vi "MissionControl2017.vi"() -> ()   [LabVIEW 2015, in "MissionControl2017.lvlib"]
uses:
  MissionControl2017.lvlib
  PathfindingSettings.ctl
  MovementSettings.ctl
  PathCostWeights.ctl
  IntermediatePositionGrids.ctl
  <vilib>/Utility/miscctls.llb/LVPoint32TypeDef.ctl
  LocalizationStatus.ctl
  <vilib>/Utility/miscctls.llb/LVBoundsTypeDef.ctl
  Vector.ctl
  PathOfMoves.ctl
  Move.ctl
  Overlord2017.lvlib
  Navigation2017.lvlib
  Navigation2017-util.lvlib
panel:
  in  "reset timer":bool
  out "millisecond timer value":u32
  in  "Turning Width (used in movement control)":dbl(slide)=0.1318325449365179 scale=0.05..0.5
  out "Waveform Chart 2":dbl(graph)=0.5
  out "Waveform Chart":dbl(graph)=0.5
  out "Motor PWM XY Graph":cluster{"X":dbl, "Y":dbl}[](graph)
  out "Position at Start of Pathfinding Calculation":T1={"x"=2.4736536245406993, "y"=1.8255455643190823, "angle"=3.0398193796851833, "valid"=TRUE, "lastUpdatedTime"=1416276.0}
  out "Current Localization Status (As Drawn Above)":T1={"x"=2.723915333589265, "y"=2.6113036938119802, "angle"=2.982809442272849, "valid"=TRUE, "lastUpdatedTime"=538657016.0}
  in  "Debug Mining":bool=TRUE
  in  "Debug Wheel Motors":bool
  out "navDebugBotSpin":dbl=1.1780972450961724
  out "y (m)":dbl=0.0073828125
  out "x (m)":dbl=3.51288
  in  "Debug Localization - Mouse":bool
  out "Mouse Wheel Sum":dbl
  out "Mouse Wheel Delta":i32
  out "Mouse Down Button":u16=1
  out "Mouse Coords":T2={"Horizontal"=524, "Vertical"=1}
  out "Mouse Down Coords":T2={"Horizontal"=778, "Vertical"=441}
  out "CurrMiningRun":i16(slide)=2 scale=0.0..3.0
  out "CurrStage":string="Moving to Mining Area"
  out "UsedDesperation":bool
  out "SpecifyingEndAngle":bool
  out "NextPointIsDestination":bool
  out "CurrNavStage":string="Waiting for localization..."
  out "FPS Indicator":bool
  in  "Pathfinding Settings":T3={"Movement Settings"={"Arrival Tolerance (m)"=0.01, "Closeness Threshold (m)"=0.5, "Pit Obstacle Radius (m)"=0.5, "Pit Locations"=[]}, "Dead Zone"=0.75, "Max Moves"=2.0, "Move Segment Length (m)"=0.2, "Path Cost Weights"={"Length Weight"=1.0, "Angle Weight"=0.0, "Angle Error Weight"=1000.0, "Angle Error Threshold"=0.314, "Per Move Penalty"=0.05, "Closeness Weight"=100.0, "Too Short Penalty"=100.0, "Too Short Threshold"=1.5}, "Desperation - Reduction Per Attempt (Ratio)"=0.9, "Desperation - Max Attempts"=1, "Log All Move Points"=TRUE, "Intermediate Position Grids"=[{"x1"=0.0, "x2"=1.75, "resolution"=0.15}, {"x1"=1.75, "x2"=7.38, "resolution"=0.4}]}
  out "Arena Pixel Size":i16[](array[numeric])=[1000, 512]
  out "Arena Control":picture
  # "NOTE: Open and pin\n\nMineOrDumpBlocking.vi\nand\nSetWheelMotorPWM.vi\n\nalongside when debugging."
  # "(Spin robot with arrow keys)"
  # "To toggle localization debugging:\n- Flip this switch <---\n- Set the Project Property -> Conditional Compilation Property\n\"DISCONNECT_LOCALIZATION\" to True or False"
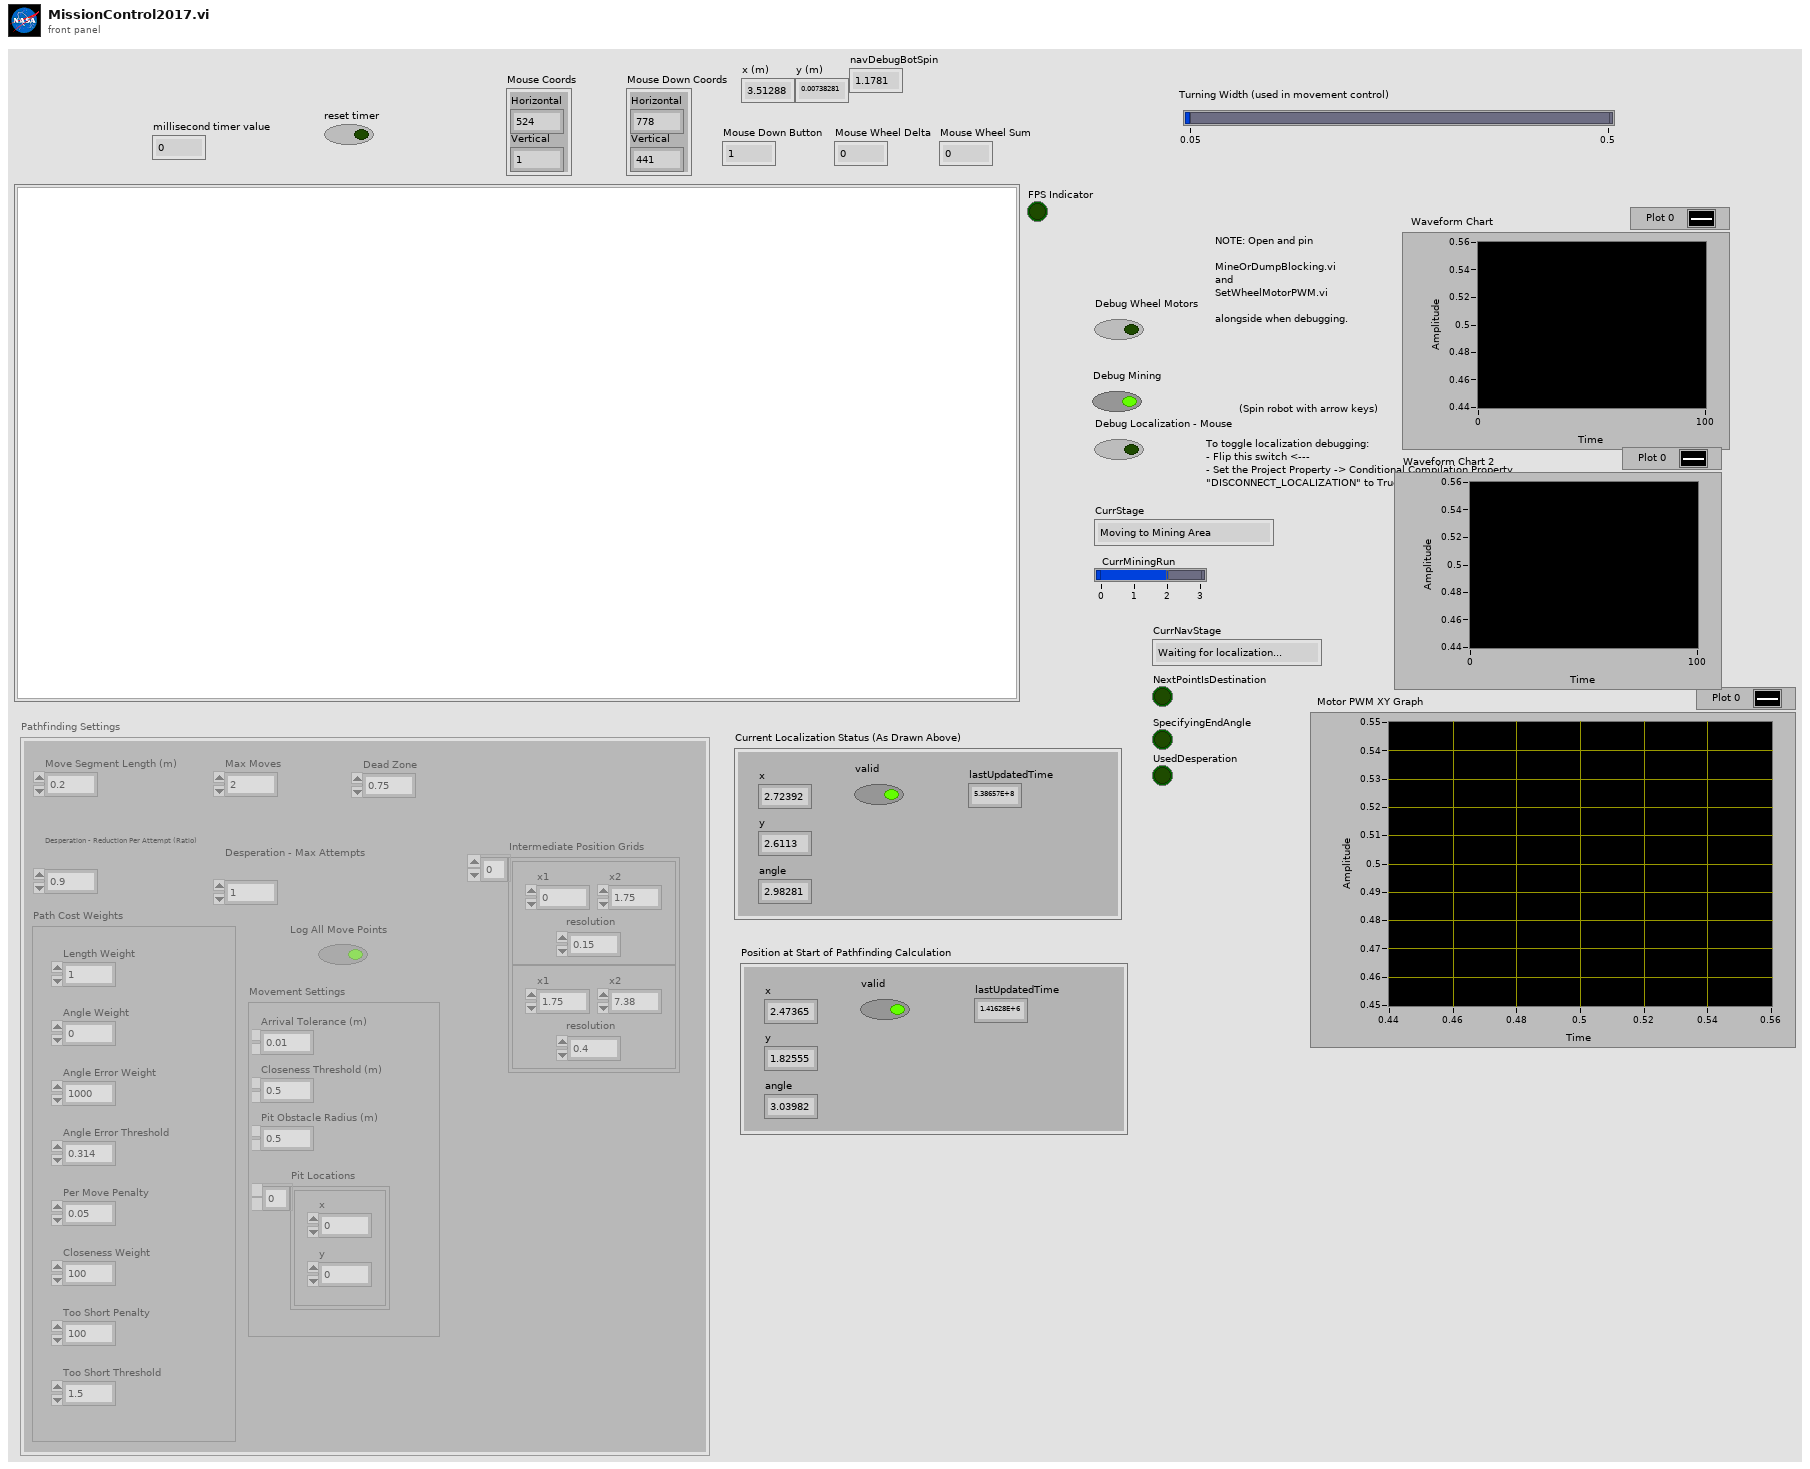
[diagram p1: front panel]
types:
  T1 = typedef "LocalizationStatus.ctl" = cluster{"x":dbl, "y":dbl, "angle":dbl, "valid":bool, "lastUpdatedTime":dbl}
  T2 = typedef "LVPoint32TypeDef.ctl" = cluster{"Horizontal":i32, "Vertical":i32}
  T3 = typedef "Navigation2017.lvlib/PathfindingSettings.ctl" = cluster{"Movement Settings":T4, "Dead Zone":dbl, "Max Moves":dbl, "Move Segment Length (m)":dbl, "Path Cost Weights":T5, "Desperation - Reduction Per Attempt (Ratio)":dbl, "Desperation - Max Attempts":i16, "Log All Move Points":bool, "Intermediate Position Grids":T6}
  T4 = typedef "Navigation2017.lvlib/MovementSettings.ctl" = cluster{"Arrival Tolerance (m)":dbl, "Closeness Threshold (m)":dbl, "Pit Obstacle Radius (m)":dbl, "Pit Locations":cluster{"x":dbl, "y":dbl}[]}
  T5 = typedef "Navigation2017.lvlib/PathCostWeights.ctl" = cluster{"Length Weight":dbl, "Angle Weight":dbl, "Angle Error Weight":dbl, "Angle Error Threshold":dbl, "Per Move Penalty":dbl, "Closeness Weight":dbl, "Too Short Penalty":dbl, "Too Short Threshold":dbl}
  T6 = typedef "Navigation2017.lvlib/IntermediatePositionGrids.ctl" = cluster{"x1":dbl, "x2":dbl, "resolution":dbl}[]
  T7 = typedef "LVBoundsTypeDef.ctl" = cluster{"Width":u32, "Height":u32}
  T8 = typedef "eventvkey.ctl" = enum16{"ASCII", "Enter", "Return", "Shift", "Ctrl", "Alt", "Cmd", "Opt", "Caps", "NumLock", "Clear", "Break", "Up", "Down", "Left", "Right", "Insert", "Delete", "Home", "End", "PageUp", "PageDown", "Escape", "Help", "Pause", "ScrollLock", "F1", "F2", "F3", "F4", "F5", "F6", "F7", "F8", "F9", "F10", "F11", "F12", "F13", "F14", "F15", "F16", "F17", "F18", "F19", "F20", "F21", "F22", "F23", "F24", "Play", "VolumeUp", "VolumeDown", "Mute", "Two Byte Char"}
  T9 = typedef "imagedata.ctl" = cluster{"image type":i32, "image depth":i32, "image":u8[], "mask":u8[], "colors":u32[], "Rectangle":cluster{"left":i16, "top":i16, "right":i16, "bottom":i16}}
  T10 = typedef "Navigation2017.lvlib/Vector.ctl" = cluster{"x":dbl, "y":dbl, "angle":dbl}
  T11 = cluster{"Width":u16, "Style":enum32{"Solid", "Dash", "Dot", "DashDot", "DashDotDot"}}
  T12 = typedef "Navigation2017.lvlib/PathOfMoves.ctl" = cluster{"Dest Angle Error":dbl, "Dest Angle Considered":bool, "Moves":T13[]}
  T13 = typedef "Navigation2017.lvlib/Move.ctl" = cluster{"Did Reach Dest":bool, "Did Collide":bool, "Sum of Angle Changes (rad)":dbl, "Move Length (m)":dbl, "Closeness Sum":dbl, "Positions Along Move":T10[], "Moved Fwd":bool}
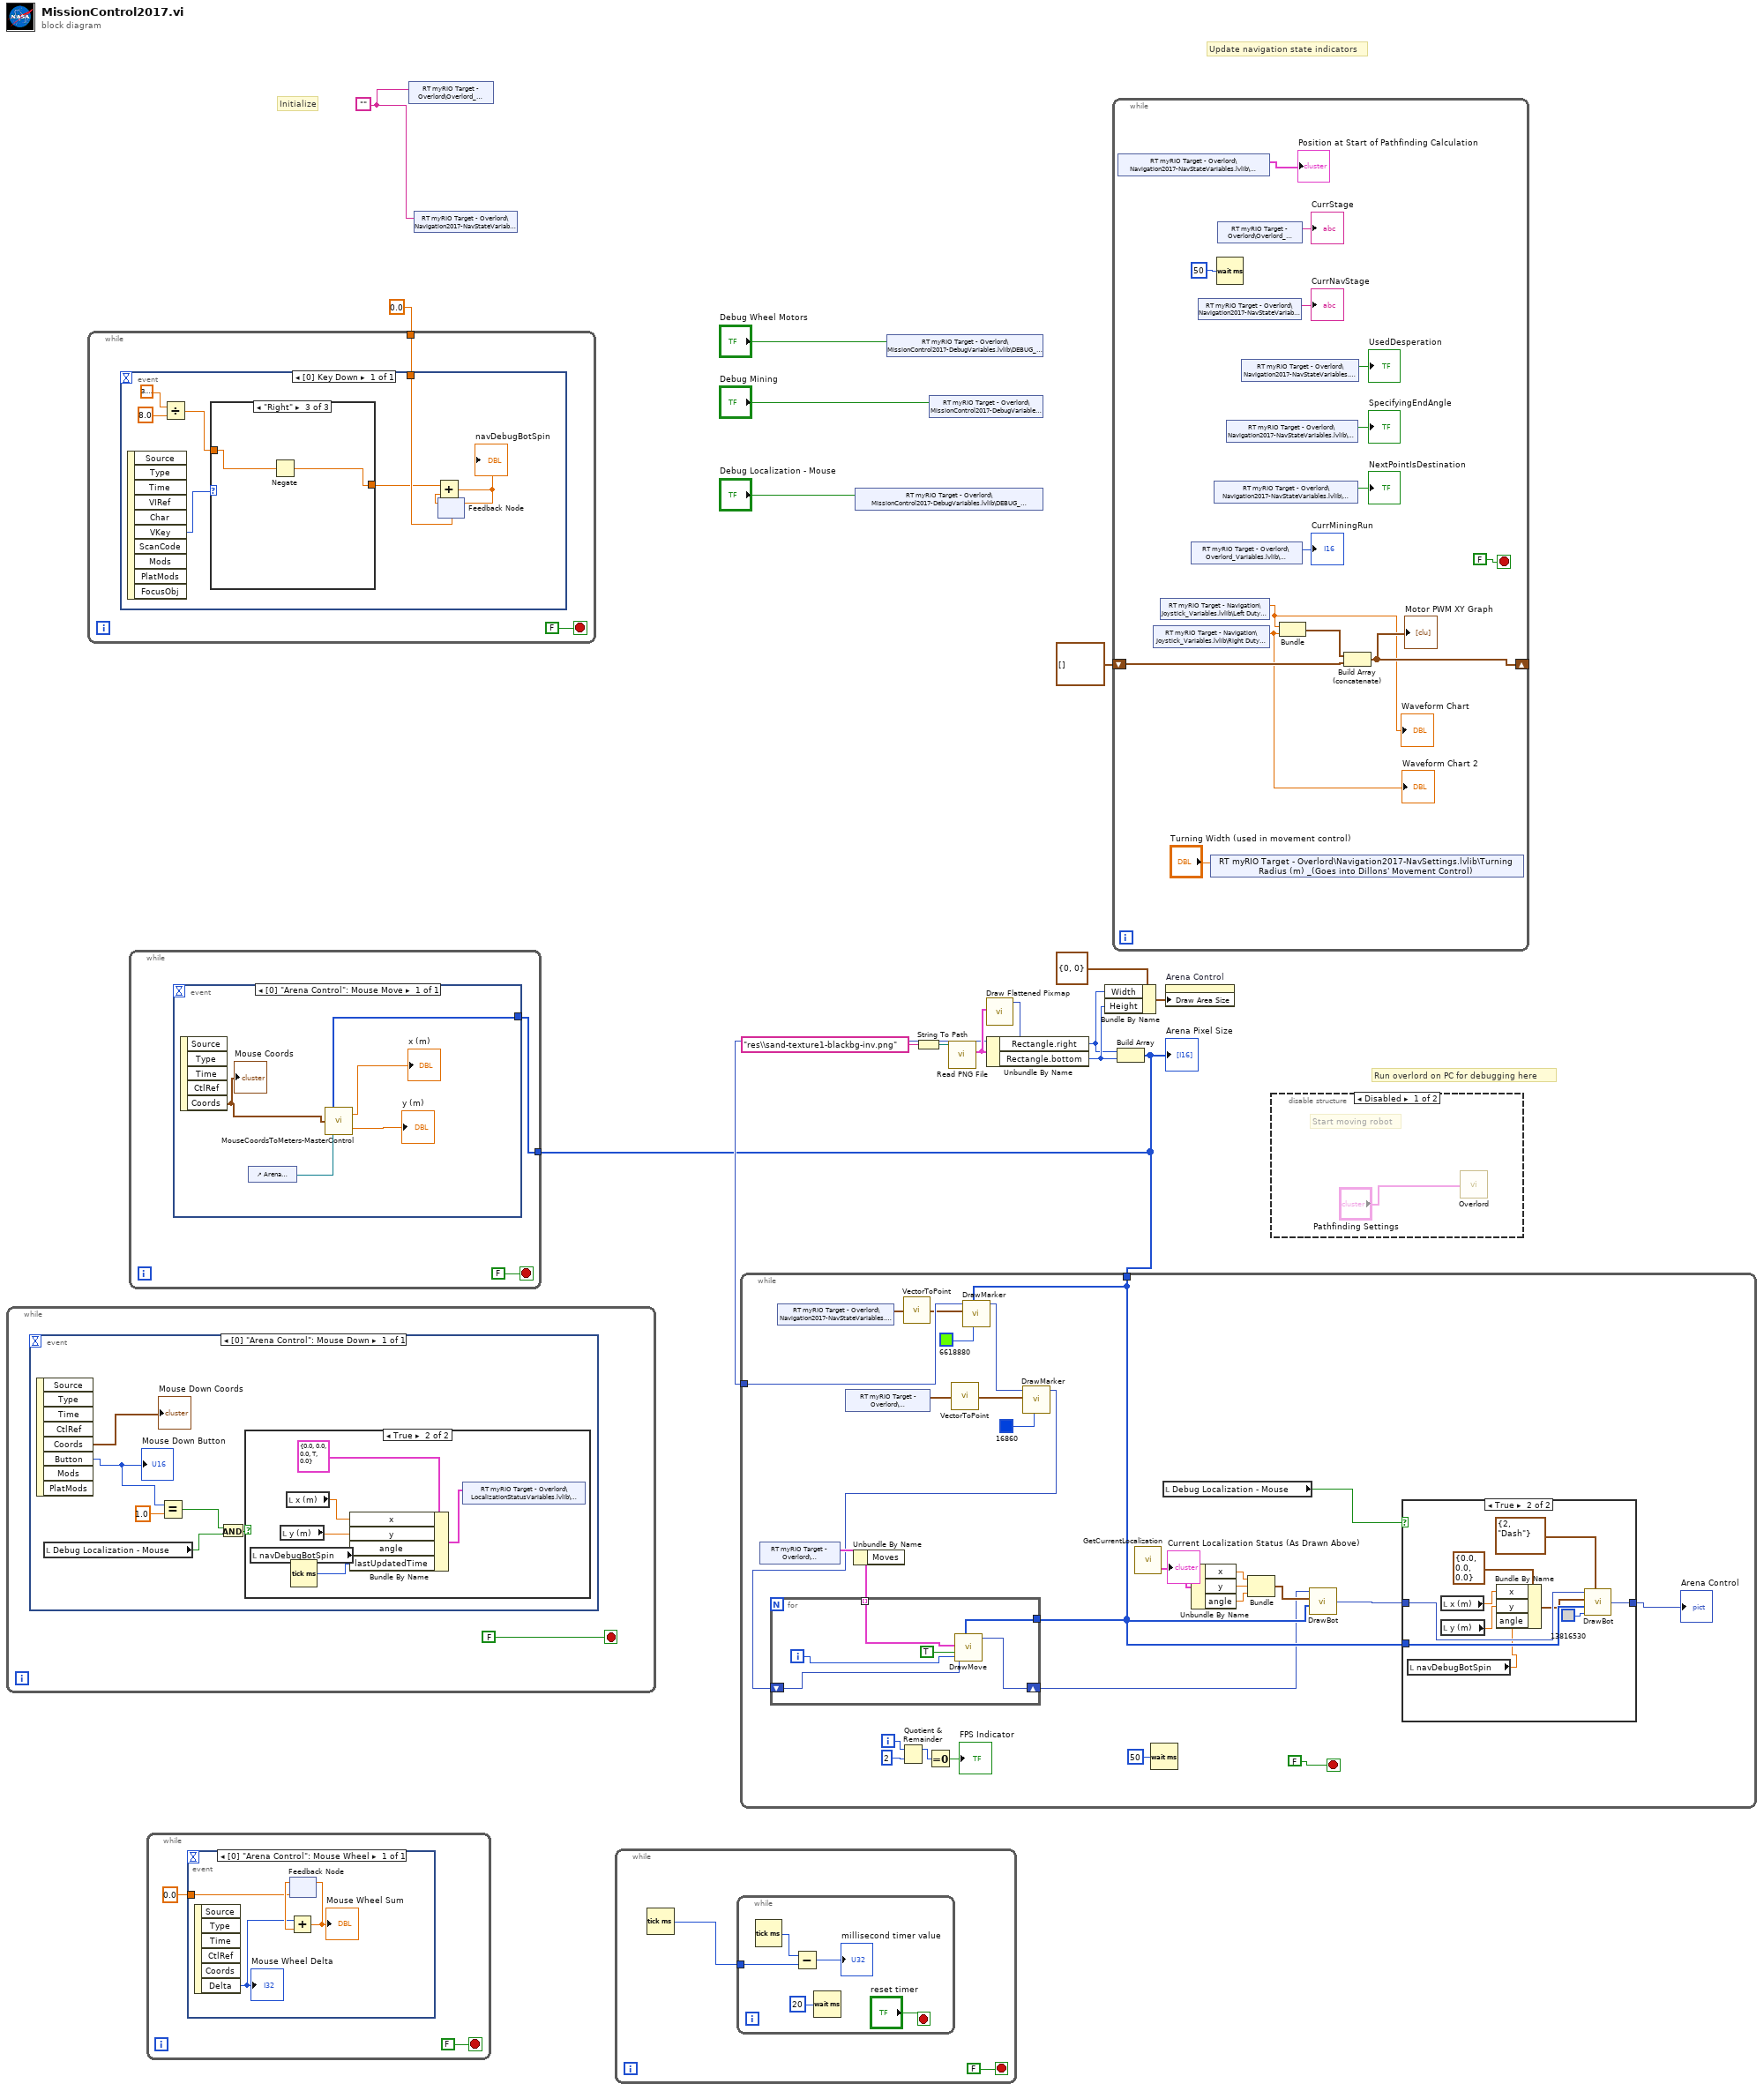
[diagram p0: block diagram]
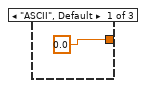
[diagram p3: hidden frame]
diagram:
  w5 = ""
  # "Run overlord on PC for debugging here"
  # "Initialize"
  # "Update navigation state indicators"
  n1 = while {
    stop <- FALSE stop-if-true
    n2 = event shown="[0] \"Arena Control\": Mouse Down" {
      selector: _ -> [_]
      dyn-events: _ -> [_]
      timeout: _ -> [_]
      event "Arena Control": Mouse Down {
        n3 = event-data() -> ("Coords"=→"Mouse Down Coords":T2, "Button"=w20:u16)  [unwired: 1 in, 6 out]
        "Mouse Down Button" <- w20
        n4 = local read "Debug Localization - Mouse"() -> (w19:bool)
        n5 = Equal?(x=w20, y=1.0) -> (x = y?=w18:bool)
        n6 = And(x=w18, y=w19) -> (x .and. y?=w17:bool)
        n7 = case shown="True" w17 {
          frame False {
          }
          frame True {
            n8 = local read "navDebugBotSpin"() -> (w23:dbl)
            n9 = local read "y (m)"() -> (w24:dbl)
            n10 = local read "x (m)"() -> (w25:dbl)
            n11 = Tick Count (ms)() -> (millisecond timer value=w26:u32)
            n12 = Bundle By Name(cluster=T1 {"x"=0.0, "y"=0.0, "angle"=0.0, "valid"=TRUE, "lastUpdatedTime"=0.0} ("Localization Status"), "x"=w25, "y"=w24, "angle"=w23, "lastUpdatedTime"=w26) -> (w27:T1)
            n13 = shared-variable "RT myRIO Target - Overlord\\LocalizationStatusVariables.lvlib\\LocalizationStatus"(w27) -> ()  [unwired: 1 in, 1 out]
          }
        }
      }
    }
  }
  n14 = while {
    tunnel: 0.0 -> [w29]
    stop <- FALSE stop-if-true
    n15 = event shown="[0] Key Down" {
      selector: _ -> [_]
      dyn-events: _ -> [_]
      timeout: _ -> [_]
      tunnel: w29 -> [w35]
      event Key Down {
        n16 = event-data() -> ("VKey"=w38:T8)  [unwired: 1 in, 9 out]
        n17 = Divide(x=3.141592653589793, y=8.0) -> (x/y=w31:dbl)
        n18 = case shown="\"Right\"" w38 {
          tunnel: [0.0 w40 w41] -> w34
          tunnel: w31 -> [_ w40 w42]
          frame "ASCII", Default {
          }
          frame "Left" {
          }
          frame "Right" {
            n19 = Negate(x=w42) -> (-x=w41:dbl)
          }
        }
        n20 = feedback #1(w35) -> (w36:dbl)
        n21 = Add(x=w34, y=w36) -> (x+y=w37:dbl)
        "navDebugBotSpin" <- w37
        n22 = feedback-in #1(w37) -> ()
      }
    }
  }
  n23 = while {
    stop <- FALSE stop-if-true
    n24 = event shown="[0] \"Arena Control\": Mouse Wheel" {
      selector: _ -> [_]
      dyn-events: _ -> [_]
      timeout: _ -> [_]
      tunnel: 0.0 -> [w46]
      event "Arena Control": Mouse Wheel {
        n25 = event-data() -> ("Delta"=w45:i32)  [unwired: 1 in, 5 out]
        "Mouse Wheel Delta" <- w45
        n26 = feedback #2(w46) -> (w47:dbl)
        n27 = Add(x=w45, y=w47) -> (x+y=w48:dbl)
        "Mouse Wheel Sum" <- w48
        n28 = feedback-in #2(w48) -> ()
      }
    }
  }
  n29 = shared-variable "RT myRIO Target - Overlord\\Overlord_Variables.lvlib\\CurrStage"(w5) -> ()  [unwired: 1 in, 1 out]
  n30 = shared-variable "RT myRIO Target - Overlord\\Navigation2017-NavStateVariables.lvlib\\CurrNavStage"(w5) -> ()  [unwired: 1 in, 1 out]
  n31 = while {
    stop <- FALSE stop-if-true
    n32 = Tick Count (ms)() -> (millisecond timer value=w50:u32)
    n33 = while {
      tunnel: w50 -> [w52]
      stop <- "reset timer" stop-if-true
      n34 = Tick Count (ms)() -> (millisecond timer value=w53:u32)
      n35 = Subtract(x=w53, y=w52) -> (x-y=→"millisecond timer value":u32)
      n36 = Wait (ms)(milliseconds to wait=u32 20) -> ()  [unwired: 1 out]
    }
  }
  n37 = shared-variable "RT myRIO Target - Overlord\\MissionControl2017-DebugVariables.lvlib\\DEBUG_LOCALIZATION_MOUSE"("Debug Localization - Mouse") -> ()  [unwired: 1 in, 1 out]
  n38 = shared-variable "RT myRIO Target - Overlord\\MissionControl2017-DebugVariables.lvlib\\DEBUG_WHEEL_MOTORS"("Debug Wheel Motors") -> ()  [unwired: 1 in, 1 out]
  n39 = String To Path(string="res\\sand-texture1-blackbg-inv.png" ("name or relative path")) -> (path=w14:path)
  n40 = shared-variable "RT myRIO Target - Overlord\\MissionControl2017-DebugVariables.lvlib\\DEBUG_BUCKET"("Debug Mining") -> ()  [unwired: 1 in, 1 out]
  n41 = call <vilib>:"Read PNG File.vi"("path to PNG file"=w14) -> ("image data"=w9:T9)  [unwired: 8 in, 2 out]
  n42 = call <vilib>:"Draw Flattened Pixmap.vi"("image data"=w9) -> ("new picture"=w8:picture)  [unwired: 8 in]
  n43 = Unbundle By Name(w9) -> ("Rectangle.right"=w11:i16, "Rectangle.bottom"=w12:i16)
  n44 = Bundle By Name(cluster=T7 {"Width"=0, "Height"=0} ("Draw Area Size"), "Width"=w11, "Height"=w12) -> (w13:T7)
  n45 = while {
    shift-right: [w59] -> _
    shift-left: cluster{"Double":dbl, "Double":dbl}[] [] -> [w60]
    stop <- FALSE stop-if-true
    n46 = shared-variable "RT myRIO Target - Overlord\\Navigation2017-NavStateVariables.lvlib\\PathfindingStartPosition"() -> (→"Position at Start of Pathfinding Calculation":T1)  [unwired: 1 in, 1 out]
    n47 = shared-variable "RT myRIO Target - Navigation\\Joystick_Variables.lvlib\\Right Duty Cycle"() -> (w58:dbl)  [unwired: 1 in, 1 out]
    "Waveform Chart 2" <- w58
    n48 = shared-variable "RT myRIO Target - Navigation\\Joystick_Variables.lvlib\\Left Duty Cycle"() -> (w57:dbl)  [unwired: 1 in, 1 out]
    "Waveform Chart" <- w57
    n49 = shared-variable "RT myRIO Target - Overlord\\Overlord_Variables.lvlib\\CurrMiningRun"() -> (→"CurrMiningRun":i16)  [unwired: 1 in, 1 out]
    n50 = shared-variable "RT myRIO Target - Overlord\\Navigation2017-NavStateVariables.lvlib\\CurrNavStage"() -> (→"CurrNavStage":string)  [unwired: 1 in, 1 out]
    n51 = shared-variable "RT myRIO Target - Overlord\\Navigation2017-NavSettings.lvlib\\Turning Radius (m) _(Goes into Dillons' Movement Control)"("Turning Width (used in movement control)") -> ()  [unwired: 1 in, 1 out]
    n52 = shared-variable "RT myRIO Target - Overlord\\Navigation2017-NavStateVariables.lvlib\\NextPointIsDestination"() -> (→"NextPointIsDestination":bool)  [unwired: 1 in, 1 out]
    n53 = Wait (ms)(milliseconds to wait=u32 50) -> ()  [unwired: 1 out]
    n54 = shared-variable "RT myRIO Target - Overlord\\Overlord_Variables.lvlib\\CurrStage"() -> (→"CurrStage":string)  [unwired: 1 in, 1 out]
    n55 = shared-variable "RT myRIO Target - Overlord\\Navigation2017-NavStateVariables.lvlib\\SpecifyingEndAngle"() -> (→"SpecifyingEndAngle":bool)  [unwired: 1 in, 1 out]
    n56 = shared-variable "RT myRIO Target - Overlord\\Navigation2017-NavStateVariables.lvlib\\UsedDesperation"() -> (→"UsedDesperation":bool)  [unwired: 1 in, 1 out]
    n57 = Bundle("Double"=w57, "Double"=w58) -> (w61:cluster{"Double":dbl, "Double":dbl})  [unwired: 1 in]
    n58 = Build Array (concatenate)(w61, w60) -> (w59:cluster{"Double":dbl, "Double":dbl}[])
    "Motor PWM XY Graph" <- w59
  }
  n59 = Build Array(w11, w12) -> (w6:i16[])
  "Arena Pixel Size" <- w6
  n60 = while {
    tunnel: w6 -> [w71]
    stop <- FALSE stop-if-true
    n61 = event shown="[0] \"Arena Control\": Mouse Move" {
      selector: _ -> [_]
      dyn-events: _ -> [_]
      timeout: _ -> [_]
      tunnel: w71 -> [w76]
      event "Arena Control": Mouse Move {
        n62 = event-data() -> ("Coords"=w77:T2)  [unwired: 1 in, 4 out]
        "Mouse Coords" <- w77
        n63 = control-ref of="Arena Control"() -> (w75:refnum<vi>)
        n64 = call "MouseCoordsToMeters-MasterControl.vi"("Picture Control Ref"=w75, "Mouse Pos"=w77, "Arena Pixel Dim"=w76) -> ("y (m)"=→"y (m)":dbl, "x (m)"=→"x (m)":dbl)
      }
    }
  }
  n65 = while {
    tunnel: w8 -> [w88]
    tunnel: w6 -> [w87]
    i -> [w103]
    stop <- FALSE stop-if-true
    n66 = shared-variable "RT myRIO Target - Overlord\\Navigation2017-NavStateVariables.lvlib\\CurrPath"() -> (w91:T12)  [unwired: 1 in, 1 out]
    n67 = shared-variable "RT myRIO Target - Overlord\\Navigation2017-NavStateVariables.lvlib\\DestinationPoint"() -> (w83:T10)  [unwired: 1 in, 1 out]
    n68 = shared-variable "RT myRIO Target - Overlord\\Navigation2017-NavStateVariables.lvlib\\NextPoint"() -> (w81:T10)  [unwired: 1 in, 1 out]
    n69 = Unbundle By Name(w91) -> ("Moves"=w90:T13[])
    n70 = Quotient & Remainder(x=w103, y=2) -> (x-y*floor(x/y)=w94:i32)  [unwired: 1 out]
    n71 = call "VectorToPoint.vi"("Vector"=w83) -> ("Point"=w84:cluster{"x":dbl, "y":dbl})
    n72 = Equal To 0?(x=w94) -> (x = 0?=→"FPS Indicator":bool)
    n73 = call "VectorToPoint.vi"("Vector"=w81) -> ("Point"=w82:cluster{"x":dbl, "y":dbl})
    n74 = call "DrawMarker.vi"("color(black)"=u32 6618880, "Arena Pixel Dim"=w87, "Cluster"=w84, "picture in"=w88) -> ("new picture"=w89:picture)  [unwired: 7 in]
    n75 = call "DrawMarker.vi"("color(black)"=u32 16860, "Cluster"=w82, "picture in"=w89) -> ("new picture"=w80:picture)  [unwired: 8 in]
    n76 = for {
      tunnel: w87 -> [w108]
      shift-right: [w109] -> w78
      shift-left: w80 -> [w110]
      tunnel: w90 -> [w106] mode=indexing
      i -> [w105]
      n77 = call "DrawMove.vi"("Arena Pixel Dim"=w108, "Move Number (optional)"=w105, "Show Vectors?"=TRUE, "Move"=w106, "picture in"=w110) -> ("picture out"=w109:picture)  [unwired: 3 in]
    }
    n78 = call "GetCurrentLocalization.vi"() -> ("Current Localization Status"=w96:T1)  [unwired: 1 out]
    "Current Localization Status (As Drawn Above)" <- w96
    n79 = Wait (ms)(milliseconds to wait=u32 50) -> ()  [unwired: 1 out]
    n80 = local read "Debug Localization - Mouse"() -> (w79:bool)
    n81 = Unbundle By Name(w96) -> ("x"=w99:dbl, "y"=w98:dbl, "angle"=w97:dbl)
    n82 = Bundle("x"=w99, "y"=w98, "angle"=w97) -> (w95:cluster{"x":dbl, "y":dbl, "angle":dbl})  [unwired: 1 in]
    n83 = call "DrawBot.vi"("picture in"=w78, "bot pos vector"=w95, "Arena Pixel Size"=w87) -> ("picture out"=w93:picture)  [unwired: 2 in]
    n84 = case shown="True" w79 {
      tunnel: w93 -> [w111 w121]
      tunnel: [w111 w120] -> w92
      tunnel: w87 -> [_ w117]
      frame False {
      }
      frame True {
        n85 = local read "navDebugBotSpin"() -> (w112:dbl)
        n86 = local read "x (m)"() -> (w114:dbl)
        n87 = local read "y (m)"() -> (w115:dbl)
        n88 = Bundle By Name(cluster=T10 {"x"=0.0, "y"=0.0, "angle"=0.0} ("Vector"), "x"=w114, "y"=w115, "angle"=w112) -> (w116:T10)
        n89 = call "DrawBot.vi"("picture in"=w121, "bot pos vector"=w116, "Arena Pixel Size"=w117, "bot color"=u32 13816530, "pen"=T11 {"Width"=2, "Style"=enum."Dash"}) -> ("picture out"=w120:picture)
      }
    }
    "Arena Control" <- w92
  }
  n90 = property on="Arena Control" class="Pict"("Draw Area Size"=w13) -> ()  [unwired: 2 in, 2 out]
  n91 = disable-structure shown="Disabled" {
    frame Disabled {
      # "Start moving robot"
      n92 = call "Overlord.vi"("Pathfinding Settings"="Pathfinding Settings") -> ()
    }
    frame Enabled {
    }
  }
